vi "get_value.vi"() -> ()   [LabVIEW 2019]
panel:
  out "spill_id_shared":i32
  in  "stop":bool
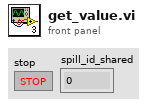
[diagram p1: front panel]
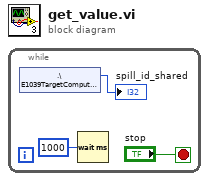
[diagram p0: block diagram]
diagram:
  n1 = while {
    stop <- "stop" stop-if-true
    n2 = shared-variable ".\\E1039TargetComputerShared.lvlib\\spill_id"() -> (→"spill_id_shared":i64)  [unwired: 1 in, 1 out]
    n3 = Wait (ms)(milliseconds to wait=u32 1000) -> ()  [unwired: 1 out]
  }
